vi "ChildClass_ReturnsValidClassInfo.vi"() -> ()   [LabVIEW 2017]
uses:
  <vilib>/addons/_JKI Toolkits/Caraya/classes/Assert/Assert Equal Value_Variant.vi
  <vilib>/addons/_JKI Toolkits/Caraya/classes/Assert/Assert Not Error.vi
  builds/TestLibrary/TestLibrary.lvlibp
  <vilib>/addons/_JKI Toolkits/Caraya/classes/Test/Test.lvclass
  <vilib>/addons/_JKI Toolkits/Caraya/classes/Assert/Assert.lvclass
panel:
  out "error out":errorcluster
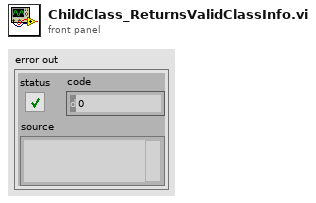
[diagram p1: front panel]
types:
  T1 = cluster{"Major":u16, "Minor":u16, "Fix":u16, "Build":u16}[]
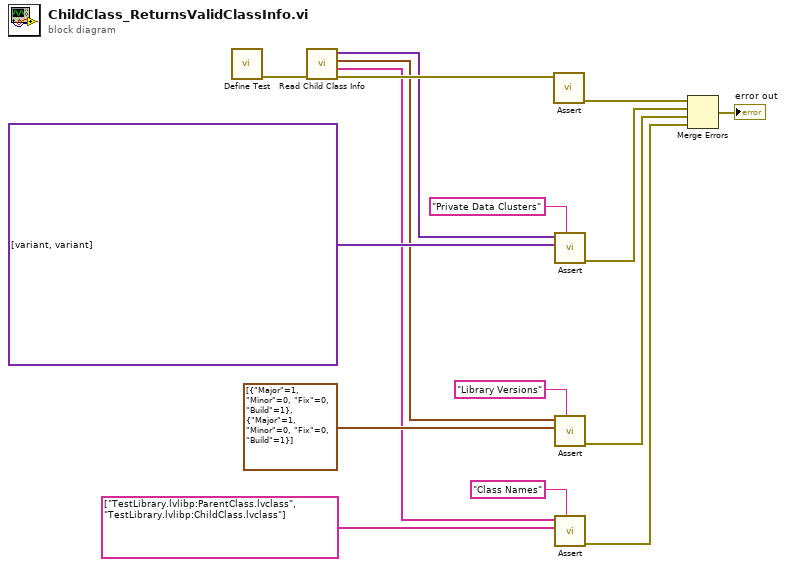
[diagram p0: block diagram]
diagram:
  n1 = call <vilib>:"Define Test.vi"() -> ("error out"=w16:errorcluster)  [unwired: 10 in, 1 out]
  n2 = call "Read Child Class Info.vi"("error in (no error)"=w16) -> ("error out"=w15:errorcluster, "Class Names"=w10:string[], "Library Versions"=w12:T1, "Private Data Clusters"=w14:variant[])  [unwired: 7 in]
  n3 = call-poly <vilib>:"Assert.vi"("Not Error?"=w15) -> ("error out"=w8:errorcluster)  [unwired: 9 in, 1 out]
  n4 = call-poly <vilib>:"Assert.vi"("Label"="Private Data Clusters", "Actual"=variant[] [variant(cluster{"Numeric":dbl} {"Numeric"=42.0}), variant(cluster{"String":string} {"String"="Hello World!"})] ("Private Data Clusters"), "Expected"=w14) -> ("error out"=w7:errorcluster)  [unwired: 7 in, 1 out]
  n5 = call-poly <vilib>:"Assert.vi"("Label"="Library Versions", "Actual"=T1 [{"Major"=1, "Minor"=0, "Fix"=0, "Build"=1}, {"Major"=1, "Minor"=0, "Fix"=0, "Build"=1}] ("Library Versions"), "Expected"=w12) -> ("error out"=w6:errorcluster)  [unwired: 7 in, 1 out]
  n6 = call-poly <vilib>:"Assert.vi"("Label"="Class Names", "Actual"=string[] ["TestLibrary.lvlibp:ParentClass.lvclass", "TestLibrary.lvlibp:ChildClass.lvclass"] ("Class Names"), "Expected"=w10) -> ("error out"=w5:errorcluster)  [unwired: 7 in, 1 out]
  n7 = Merge Errors(w8, w7, w6, w5) -> (→"error out":errorcluster)
